vi "Close Notifiers.vi"(8 "error in":errorcluster, 11 "Notifiers":T1) -> (0 "error out":errorcluster)   [LabVIEW 2014]
uses:
  Notifiers.ctl
  Message Handler Loop Notifiers.ctl
  Hardware Control/Parameter Analyzer/Parameter Analyzer Notifiers.ctl
  Hardware Control/Switching Matrix/Switching Matrix Notifiers.ctl
  Hardware Control/Stress Control/StressControl Notifiers.ctl
  Hardware Control/Spectrometer/Spectrometer Notifiers.ctl
  Hardware Control/Switches and Mirrors/SwitchesMirrors Notifiers.ctl
  Hardware Control/Camera/Camera Notifiers.ctl
  Hardware Control/XYZ Stage/XYZ Notifications.ctl
  Hardware Control/Autofocus/Autofocus Notifiers.ctl
  Measurements/Optoelectronic Measurement/Optoelectronic Notifiers.ctl
  Measurements/Save Data/SaveData Notifiers.ctl
  Measurements/Instrument Sequence/Instrument Sequence Notifiers.ctl
panel:
  # "LICENSED MATERIALS – PROPERTY OF IBM\nCopyright IBM Corp. 2016,\nALL RIGHTS RESERVED"
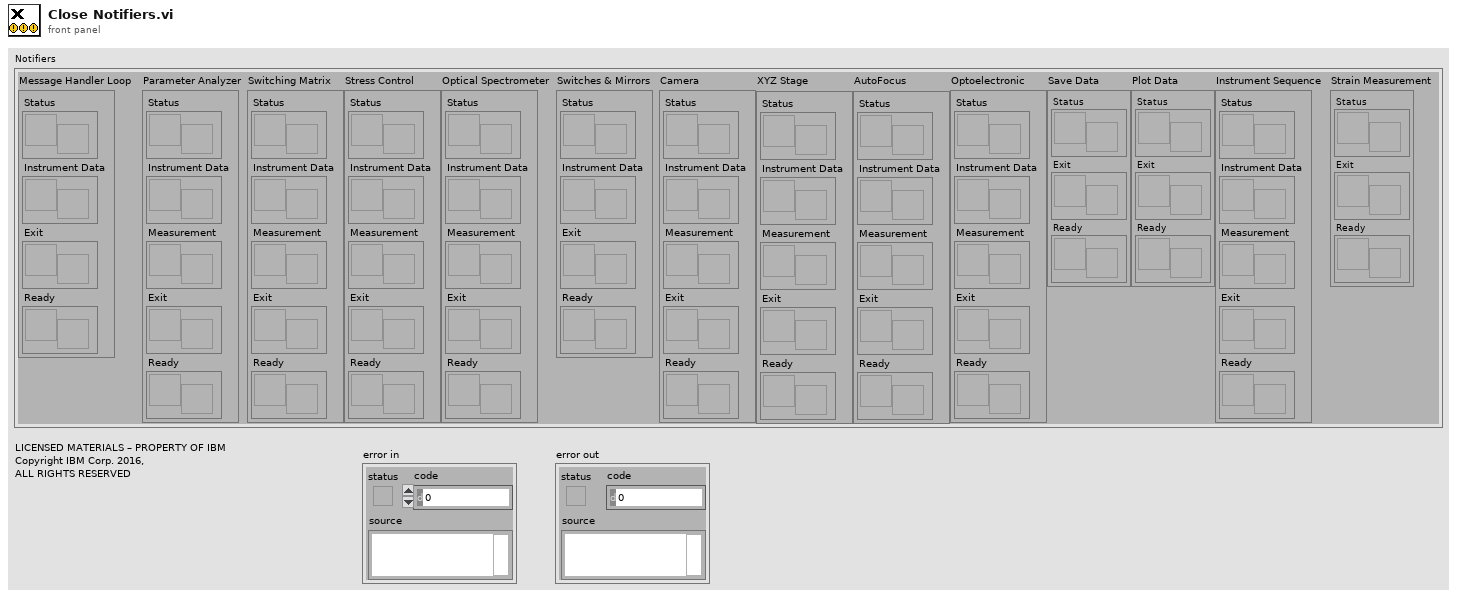
[diagram p1: front panel]
types:
  T1 = typedef "Notifiers.ctl" = cluster{"Message Handler Loop":T2, "Parameter Analyzer":T3, "Switching Matrix":T4, "Stress Control":T5, "Optical Spectrometer":T6, "Switches & Mirrors":T7, "Camera":T8, "XYZ Stage":T9, "AutoFocus":T10, "Optoelectronic":T11, "Save Data":T12, "Plot Data":T12, "Instrument Sequence":T13, "Strain Measurement":cluster{"Status":refnum<notifier>, "Exit":refnum<notifier>, "Ready":refnum<notifier>}}
  T2 = typedef "Message Handler Loop Notifiers.ctl" = cluster{"Status":refnum<notifier>, "Instrument Data":refnum<notifier>, "Exit":refnum<notifier>, "Ready":refnum<notifier>}
  T3 = typedef "Parameter Analyzer Notifiers.ctl" = cluster{"Status":refnum<notifier>, "Instrument Data":refnum<notifier>, "Measurement":refnum<notifier>, "Exit":refnum<notifier>, "Ready":refnum<notifier>}
  T4 = typedef "Switching Matrix Notifiers.ctl" = cluster{"Status":refnum<notifier>, "Instrument Data":refnum<notifier>, "Measurement":refnum<notifier>, "Exit":refnum<notifier>, "Ready":refnum<notifier>}
  T5 = typedef "StressControl Notifiers.ctl" = cluster{"Status":refnum<notifier>, "Instrument Data":refnum<notifier>, "Measurement":refnum<notifier>, "Exit":refnum<notifier>, "Ready":refnum<notifier>}
  T6 = typedef "Spectrometer Notifiers.ctl" = cluster{"Status":refnum<notifier>, "Instrument Data":refnum<notifier>, "Measurement":refnum<notifier>, "Exit":refnum<notifier>, "Ready":refnum<notifier>}
  T7 = typedef "SwitchesMirrors Notifiers.ctl" = cluster{"Status":refnum<notifier>, "Instrument Data":refnum<notifier>, "Exit":refnum<notifier>, "Ready":refnum<notifier>}
  T8 = typedef "Camera Notifiers.ctl" = cluster{"Status":refnum<notifier>, "Instrument Data":refnum<notifier>, "Measurement":refnum<notifier>, "Exit":refnum<notifier>, "Ready":refnum<notifier>}
  T9 = typedef "XYZ Notifications.ctl" = cluster{"Status":refnum<notifier>, "Instrument Data":refnum<notifier>, "Measurement":refnum<notifier>, "Exit":refnum<notifier>, "Ready":refnum<notifier>}
  T10 = typedef "Autofocus Notifiers.ctl" = cluster{"Status":refnum<notifier>, "Instrument Data":refnum<notifier>, "Measurement":refnum<notifier>, "Exit":refnum<notifier>, "Ready":refnum<notifier>}
  T11 = typedef "Optoelectronic Notifiers.ctl" = cluster{"Status":refnum<notifier>, "Instrument Data":refnum<notifier>, "Measurement":refnum<notifier>, "Exit":refnum<notifier>, "Ready":refnum<notifier>}
  T12 = typedef "SaveData Notifiers.ctl" = cluster{"Status":refnum<notifier>, "Exit":refnum<notifier>, "Ready":refnum<notifier>}
  T13 = typedef "Instrument Sequence Notifiers.ctl" = cluster{"Status":refnum<notifier>, "Instrument Data":refnum<notifier>, "Measurement":refnum<notifier>, "Exit":refnum<notifier>, "Ready":refnum<notifier>}
  T14 = cluster{"Status":refnum<notifier>, "Exit":refnum<notifier>, "Ready":refnum<notifier>}
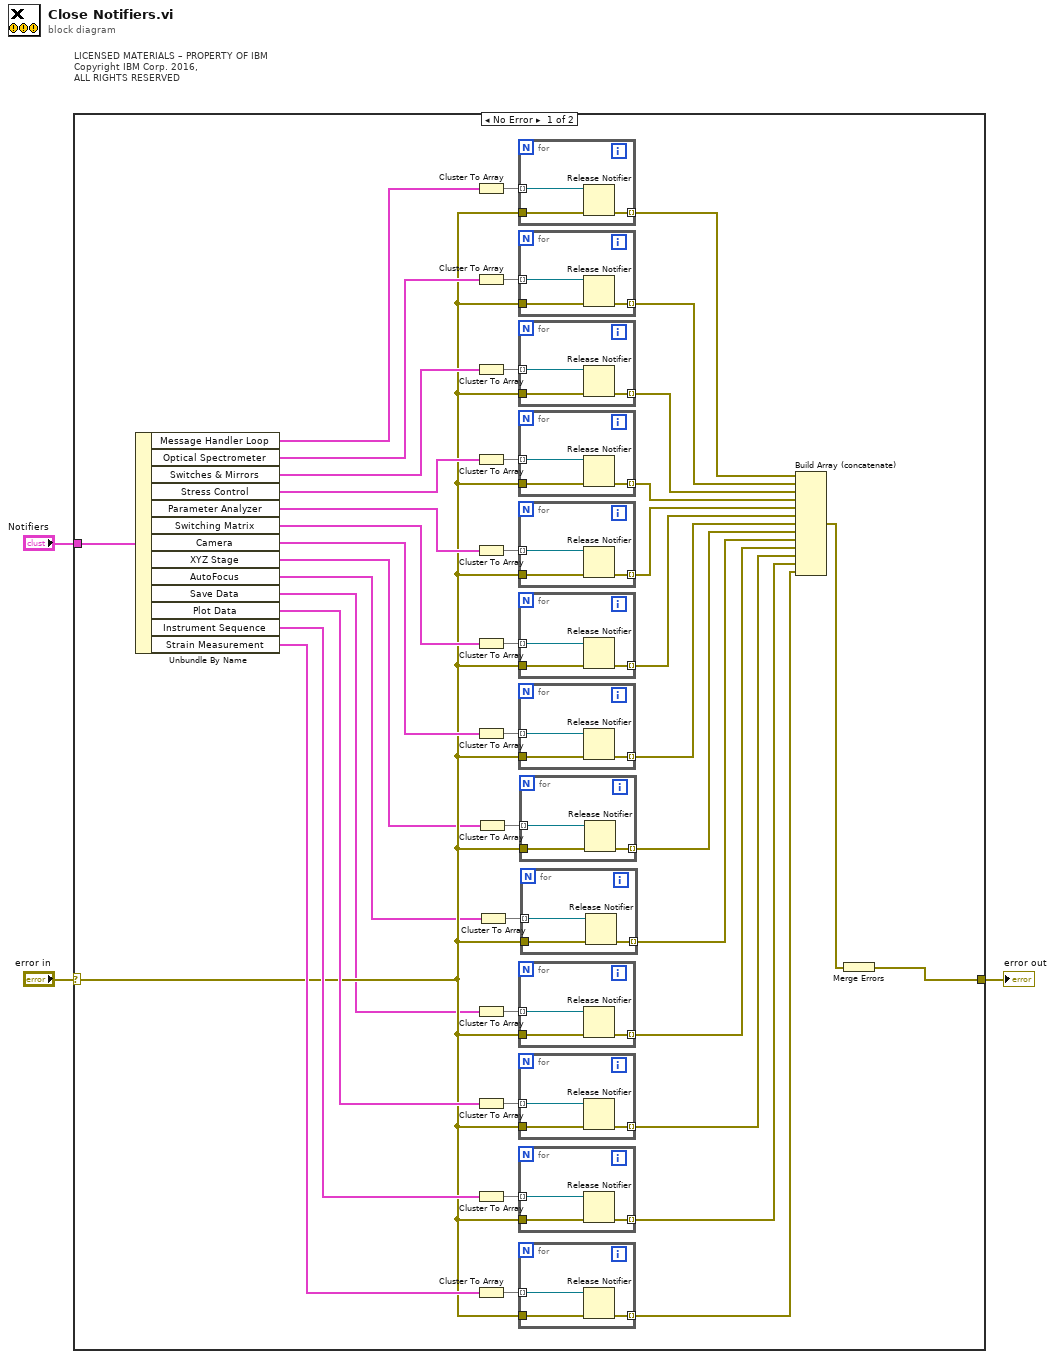
[diagram p0: block diagram]
diagram:
  # "LICENSED MATERIALS – PROPERTY OF IBM\nCopyright IBM Corp. 2016,\nALL RIGHTS RESERVED"
  n1 = case shown="No Error" "error in" {
    selector: "error in" -> [w9 w86]
    tunnel: "Notifiers" -> [w46 _]
    tunnel: [w45 w86] -> w2
    frame No Error {
      n2 = Unbundle By Name(w46) -> ("Message Handler Loop"=w32:T2, "Optical Spectrometer"=w33:T6, "Switches & Mirrors"=w34:T7, "Stress Control"=w35:T5, "Parameter Analyzer"=w36:T3, "Switching Matrix"=w37:T4, "Camera"=w24:T8, "XYZ Stage"=w4:T9, "AutoFocus"=w5:T10, "Save Data"=w6:T12, "Plot Data"=w13:T12, "Instrument Sequence"=w14:T13, "Strain Measurement"=w15:T14)
      n3 = Cluster To Array(cluster=w32) -> (array=w38:refnum<notifier>[])
      n4 = Cluster To Array(cluster=w33) -> (array=w43:refnum<notifier>[])
      n5 = Cluster To Array(cluster=w34) -> (array=w42:refnum<notifier>[])
      n6 = Cluster To Array(cluster=w35) -> (array=w41:refnum<notifier>[])
      n7 = Cluster To Array(cluster=w36) -> (array=w40:refnum<notifier>[])
      n8 = Cluster To Array(cluster=w37) -> (array=w39:refnum<notifier>[])
      n9 = Cluster To Array(cluster=w24) -> (array=w23:refnum<notifier>[])
      n10 = Cluster To Array(cluster=w6) -> (array=w22:refnum<notifier>[])
      n11 = Cluster To Array(cluster=w13) -> (array=w20:refnum<notifier>[])
      n12 = Cluster To Array(cluster=w14) -> (array=w18:refnum<notifier>[])
      n13 = Cluster To Array(cluster=w15) -> (array=w16:refnum<notifier>[])
      n14 = Cluster To Array(cluster=w4) -> (array=w11:refnum<notifier>[])
      n15 = Cluster To Array(cluster=w5) -> (array=w10:refnum<notifier>[])
      n16 = for {
        tunnel: w38 -> [w68] mode=indexing
        tunnel: w9 -> [w70]
        tunnel: [w69] -> w26 mode=indexing
        n17 = Release Notifier(notifier=w68, error in (no error)=w70) -> (error out=w69:errorcluster)  [unwired: 3 out]
      }
      n18 = for {
        tunnel: w43 -> [w83] mode=indexing
        tunnel: w9 -> [w85]
        tunnel: [w84] -> w27 mode=indexing
        n19 = Release Notifier(notifier=w83, error in (no error)=w85) -> (error out=w84:errorcluster)  [unwired: 3 out]
      }
      n20 = for {
        tunnel: w42 -> [w80] mode=indexing
        tunnel: w9 -> [w82]
        tunnel: [w81] -> w28 mode=indexing
        n21 = Release Notifier(notifier=w80, error in (no error)=w82) -> (error out=w81:errorcluster)  [unwired: 3 out]
      }
      n22 = for {
        tunnel: w41 -> [w77] mode=indexing
        tunnel: w9 -> [w79]
        tunnel: [w78] -> w29 mode=indexing
        n23 = Release Notifier(notifier=w77, error in (no error)=w79) -> (error out=w78:errorcluster)  [unwired: 3 out]
      }
      n24 = for {
        tunnel: w40 -> [w74] mode=indexing
        tunnel: w9 -> [w76]
        tunnel: [w75] -> w30 mode=indexing
        n25 = Release Notifier(notifier=w74, error in (no error)=w76) -> (error out=w75:errorcluster)  [unwired: 3 out]
      }
      n26 = for {
        tunnel: w39 -> [w71] mode=indexing
        tunnel: w9 -> [w73]
        tunnel: [w72] -> w31 mode=indexing
        n27 = Release Notifier(notifier=w71, error in (no error)=w73) -> (error out=w72:errorcluster)  [unwired: 3 out]
      }
      n28 = for {
        tunnel: w9 -> [w67]
        tunnel: [w66] -> w25 mode=indexing
        tunnel: w23 -> [w65] mode=indexing
        n29 = Release Notifier(notifier=w65, error in (no error)=w67) -> (error out=w66:errorcluster)  [unwired: 3 out]
      }
      n30 = for {
        tunnel: w9 -> [w64]
        tunnel: [w63] -> w21 mode=indexing
        tunnel: w22 -> [w62] mode=indexing
        n31 = Release Notifier(notifier=w62, error in (no error)=w64) -> (error out=w63:errorcluster)  [unwired: 3 out]
      }
      n32 = for {
        tunnel: w9 -> [w61]
        tunnel: [w60] -> w19 mode=indexing
        tunnel: w20 -> [w59] mode=indexing
        n33 = Release Notifier(notifier=w59, error in (no error)=w61) -> (error out=w60:errorcluster)  [unwired: 3 out]
      }
      n34 = for {
        tunnel: w9 -> [w58]
        tunnel: [w57] -> w17 mode=indexing
        tunnel: w18 -> [w56] mode=indexing
        n35 = Release Notifier(notifier=w56, error in (no error)=w58) -> (error out=w57:errorcluster)  [unwired: 3 out]
      }
      n36 = for {
        tunnel: w9 -> [w55]
        tunnel: [w54] -> w12 mode=indexing
        tunnel: w16 -> [w53] mode=indexing
        n37 = Release Notifier(notifier=w53, error in (no error)=w55) -> (error out=w54:errorcluster)  [unwired: 3 out]
      }
      n38 = for {
        tunnel: w9 -> [w52]
        tunnel: [w51] -> w8 mode=indexing
        tunnel: w11 -> [w50] mode=indexing
        n39 = Release Notifier(notifier=w50, error in (no error)=w52) -> (error out=w51:errorcluster)  [unwired: 3 out]
      }
      n40 = for {
        tunnel: w9 -> [w49]
        tunnel: [w48] -> w7 mode=indexing
        tunnel: w10 -> [w47] mode=indexing
        n41 = Release Notifier(notifier=w47, error in (no error)=w49) -> (error out=w48:errorcluster)  [unwired: 3 out]
      }
      n42 = Build Array (concatenate)(w26, w27, w28, w29, w30, w31, w25, w8, w7, w21, w19, w17, w12) -> (w44:errorcluster[])
      n43 = Merge Errors(w44) -> (w45:errorcluster)
    }
    frame Error {
    }
  }
  "error out" <- w2
